vi "DiffDrivePoseEst_SetVisionMeasurementStdDevs.vi"(10 "VisionMeasurementStdDevs":T1, 11 "in DiffDrivePoseEstimate":T2={"M_VisionDiscR"=[], "m_nominal_dT"=0.0, "m_PrevTime_Sec"=0.0, "m_GyroOffset"={"VALUE"=0.0, "COS"=1.0, "SIN"=0.0}, "m_PrevAngle"={"VALUE"=0.0, "COS"=1.0, "SIN"=0.0}, "StartLeftEnc_M"=0.0, "StartRightEnc_M"=0.0, "m_Observer"={"m_P"=[], "m_xHat"=[], "States"=0, "Outputs"=0, "m_ContR"=[], "m_ContQ"=[], "m_SigmasF"=[], "m_dT_Sec"=0.0, "MERWE_SCALED_SIGMA_PTS"={"m_Wm"=[], "States"=0, "Alpha"=0.0, "m_Wc"=[], "Kappa"=0}, "meanFuncX"=refnum, "meanFuncY"=refnum, "residualFuncX"=refnum, "residualFuncY"=refnum, "addFuncX"=refnum, "addFuncXExtra"=variant, "residualFuncYExtra"=variant, "residualFuncXExtra"=variant, "MeanFuncYExtra"=variant, "MeanFuncXExtra"=variant, "Inputs"=0}, "m_latencyCompensator"={"m_pastObserverSnapshots "=[]}} {"m_PrevAngle"."SIN" format="%13.4f"; "m_PrevAngle"."COS" format="%13.4f"; "m_PrevAngle"."VALUE" format="%13.4f"; "m_GyroOffset"."SIN" format="%13.4f"; "m_GyroOffset"."COS" format="%13.4f"; "m_GyroOffset"."VALUE" format="%13.4f"}) -> (0 "Size Coerced":bool, 3 "Out DiffDrivePoseEstimate":T2={"M_VisionDiscR"=[], "m_nominal_dT"=0.0, "m_PrevTime_Sec"=0.0, "m_GyroOffset"={"VALUE"=0.0, "COS"=1.0, "SIN"=0.0}, "m_PrevAngle"={"VALUE"=0.0, "COS"=1.0, "SIN"=0.0}, "StartLeftEnc_M"=0.0, "StartRightEnc_M"=0.0, "m_Observer"={"m_P"=[], "m_xHat"=[], "States"=0, "Outputs"=0, "m_ContR"=[], "m_ContQ"=[], "m_SigmasF"=[], "m_dT_Sec"=0.0, "MERWE_SCALED_SIGMA_PTS"={"m_Wm"=[], "States"=0, "Alpha"=0.0, "m_Wc"=[], "Kappa"=0}, "meanFuncX"=refnum, "meanFuncY"=refnum, "residualFuncX"=refnum, "residualFuncY"=refnum, "addFuncX"=refnum, "addFuncXExtra"=variant, "residualFuncYExtra"=variant, "residualFuncXExtra"=variant, "MeanFuncYExtra"=variant, "MeanFuncXExtra"=variant, "Inputs"=0}, "m_latencyCompensator"={"m_pastObserverSnapshots "=[]}} {"m_PrevAngle"."SIN" format="%13.4f"; "m_PrevAngle"."COS" format="%13.4f"; "m_PrevAngle"."VALUE" format="%13.4f"; "m_GyroOffset"."SIN" format="%13.4f"; "m_GyroOffset"."COS" format="%13.4f"; "m_GyroOffset"."VALUE" format="%13.4f"})   [LabVIEW 2019, in "Trajectory_Library.lvlib"]
doc: "Sets the pose estimator's trust of global measurements. This might be used to change trust in vision measurements after the autonomous period, or to change trust as distance to a vision target increases.\n\nInputs:\n - inDiffDrivePoseEst -- System data cluster \n - visionMeasurementStdDevs -- Standard deviations of the vision measurements. Increase these numbers to trust global measurements from vision less. This matrix is in the form [x, y, theta]?, with units in meters and radians.\n\nOutputs:\n - outDiffDrivePoseEst -- System data cluster \n - error -- A value of TRUE indicates an unexpected error occured."
uses:
  Trajectory_Library.lvlib
  DIFF_DRIVE_POSE_EST.ctl
  <vilib>/Analysis/Matrix/Datatypes/RealMatrix.ctl
  ROTATION2D.ctl
  UNSCENTED_KALMAN_FILTER.ctl
  MERWE_SCALED_SIGMA_PTS.ctl
  CALLBACK_FUNC_TYPE.ctl
  KALMAN_FILTER_LATENCY_COMP.ctl
  OBSERVER_SNAP_LIST_ITEM.ctl
  OBSERVER_SNAPSHOT.ctl
  MatBuilder_Create.vi
  MatrixHelper_CoerceSize.vi
  <vilib>/Analysis/Matrix/NI_Matrix.lvlib
panel:
  # "<3, 1>"
  # "<3, 3>"
  # "<Statess,1>"
  # "<States, States>"
  # "<Inputs, 1>"
  # "<Outputs,  1>"
  # "State Estimate <Statess,1>"
  # "<States, States>"
  # "<States, ?>"
  # "<Statess,  States>"
  # "<Outputs, Outputs>"
  # "<?, 1>"
  # "<?, 1>"
  # "<3, 3>"
  # "<Statess,1>"
  # "<States, States>"
  # "<Inputs, 1>"
  # "<Outputs,  1>"
  # "State Estimate <Statess,1>"
  # "<States, States>"
  # "<States, ?>"
  # "<Statess,  States>"
  # "<Outputs, Outputs>"
  # "<?, 1>"
  # "<?, 1>"
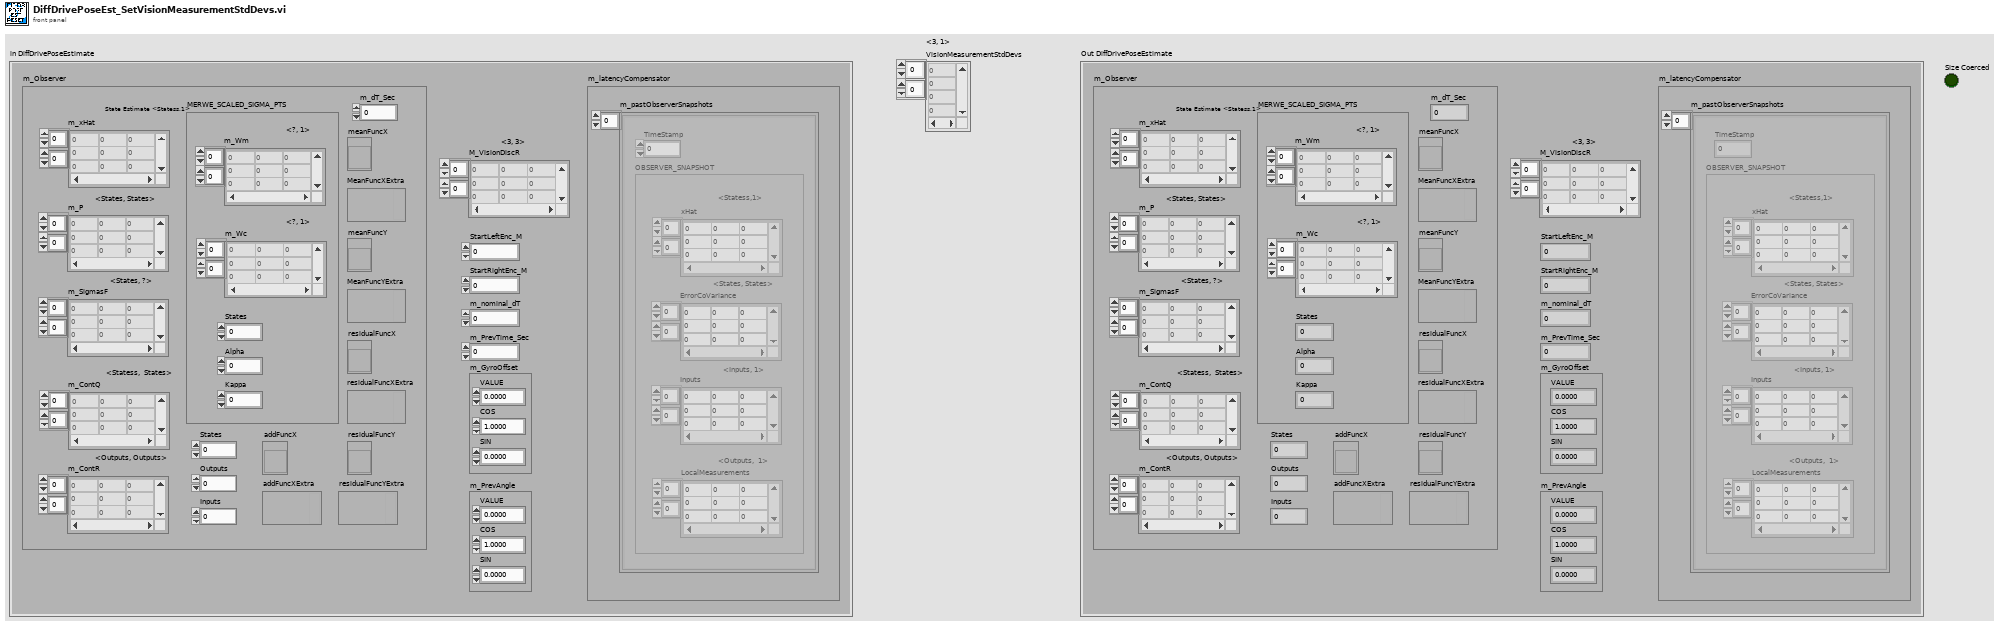
[diagram p1: front panel]
types:
  T1 = typedef "NI_Matrix.lvlib/RealMatrix.ctl" = dbl[][]
  T2 = typedef "Trajectory_Library.lvlib/DIFF_DRIVE_POSE_EST.ctl" = cluster{"M_VisionDiscR":T1, "m_nominal_dT":dbl, "m_PrevTime_Sec":dbl, "m_GyroOffset":T3, "m_PrevAngle":T3, "StartLeftEnc_M":dbl, "StartRightEnc_M":dbl, "m_Observer":T4, "m_latencyCompensator":T7}
  T3 = typedef "Trajectory_Library.lvlib/ROTATION2D.ctl" = cluster{"VALUE":dbl, "COS":dbl, "SIN":dbl}
  T4 = typedef "Trajectory_Library.lvlib/UNSCENTED_KALMAN_FILTER.ctl" = cluster{"m_P":T1, "m_xHat":T1, "States":i32, "Outputs":i32, "m_ContR":T1, "m_ContQ":T1, "m_SigmasF":T1, "m_dT_Sec":dbl, "MERWE_SCALED_SIGMA_PTS":T5, "meanFuncX":T6, "meanFuncY":T6, "residualFuncX":T6, "residualFuncY":T6, "addFuncX":T6, "addFuncXExtra":variant, "residualFuncYExtra":variant, "residualFuncXExtra":variant, "MeanFuncYExtra":variant, "MeanFuncXExtra":variant, "Inputs":i32}
  T5 = typedef "Trajectory_Library.lvlib/MERWE_SCALED_SIGMA_PTS.ctl" = cluster{"m_Wm":T1, "States":i32, "Alpha":dbl, "m_Wc":T1, "Kappa":i32}
  T6 = typedef "Trajectory_Library.lvlib/CALLBACK_FUNC_TYPE.ctl" = refnum<vi>
  T7 = typedef "Trajectory_Library.lvlib/KALMAN_FILTER_LATENCY_COMP.ctl" = cluster{"m_pastObserverSnapshots ":T8[]}
  T8 = typedef "Trajectory_Library.lvlib/OBSERVER_SNAP_LIST_ITEM.ctl" = cluster{"TimeStamp":dbl, "OBSERVER_SNAPSHOT":T9}
  T9 = typedef "Trajectory_Library.lvlib/OBSERVER_SNAPSHOT.ctl" = cluster{"ErrorCoVariance":T1, "xHat":T1, "LocalMeasurements":T1, "Inputs":T1}
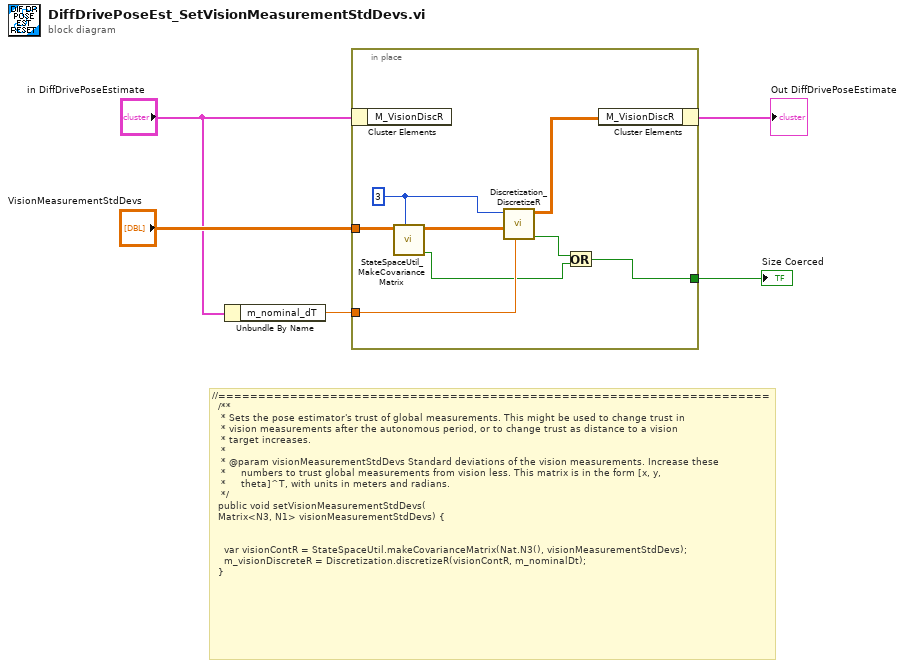
[diagram p0: block diagram]
diagram:
  # "//=====================================================================\n  /**\n   * Sets the pose estimator's trust of global measurements. This might be used to change trust in\n   * vision measurements after the autonomous period, or to change trust as distance to a vision\n   * target increases.\n   *\n   * @param visionMeasurementStdDevs Standard deviations of the vision measurements. Increase these\n   *     numbers to trust global measurements from vision less. This matrix is in the form [x, y,\n   *     theta]^T, with units in meters and radians.\n   */\n  public void setVisionMeasurementStdDevs(\n\t\tMatrix<N3, N1> visionMeasurementStdDevs) {\n\n\n    var visionContR = StateSpaceUtil.makeCovarianceMatrix(Nat.N3(), visionMeasurementStdDevs);\n    m_visionDiscreteR = Discretization.discretizeR(visionContR, m_nominalDt);\n  }"
  n1 = Unbundle By Name("in DiffDrivePoseEstimate") -> ("m_nominal_dT"=w2:dbl)
  n2 = in-place {
    in-place-border: "VisionMeasurementStdDevs" -> [w13]
    in-place-border: w2 -> [w11]
    in-place-border: [w6] -> w1
    w10 = 3 ("States")
    n3 = in-place-cluster #1("in DiffDrivePoseEstimate") -> ()  [unwired: 1 out]
    n4 = call "StateSpaceUtil_MakeCovarianceMatrix.vi"("States"=w10, "StdDevs"=w13) -> ("Size Coerced"=w8:bool, "Covariance Matrix"=w12:T1)  [unwired: 8 in]
    n5 = call "Discretization_DiscretizeR.vi"("dT_Seconds"=w11, "ContR"=w12, "Outputs"=w10) -> ("Size Coerced"=w7:bool, "DiscR"=w9:T1)  [unwired: 7 in]
    n6 = Or(x=w7, y=w8) -> (x .or. y?=w6:bool)
    n7 = in-place-cluster #1("M_VisionDiscR"=w9) -> (→"Out DiffDrivePoseEstimate":T2)
  }
  "Size Coerced" <- w1
